vi "rotina de aquisição dos dados de caracterização.vi"() -> ()   [LabVIEW 2011]
uses:
  <vilib>/express/express analysis/Spectral/XNode/ExpressSpectralMeasurementsBlockNode.xnode
  <vilib>/express/express analysis/Spectral/Block/exnSpectralBlock spectral measurements power poly.vi
  <vilib>/express/express analysis/Spectral/Block/exnSpectralBlock spectral measurements power DDT.vi
  <vilib>/express/express analysis/Spectral/Block/exnSpectralBlock spectral measurements power WFM.vi
panel:
  out "Power Spectrum":cluster{"f0":dbl, "df":dbl, "magnitude":dbl[]}(graph)
  in  "Upper Cut-Off":dbl=65.0
  out "Waveform Graph":dynamicdata(graph)
  in  "Frequência de Corte (Hz)":dbl=60.0 caption="Lower Cut-Off"
  out "Gráfico - tempo real/sinal bruto":dbl[](graph) caption="Gráfico - tempo real/bruto"
  in  "stop":bool
  out "Gráfico - tempo real/sinal filtrado":dbl[](graph) caption="Gráfico - tempo real/filtrado"
  out "Gráfico 2":waveform(dbl)(graph)
  in  "Parar programa":bool
  in  "OK Button":bool
  out "direito":dbl
  out "esquerdo":dbl
  # "PROGRAMA DE AQUISIÇÃO DE SINAL PARA CARACTERIZAÇÃO"
  # "SINAL AQUISITADO EM TEMPO REAL"
  # "SINAL A SER GRAVADO PARA PROCESSAMENTO"
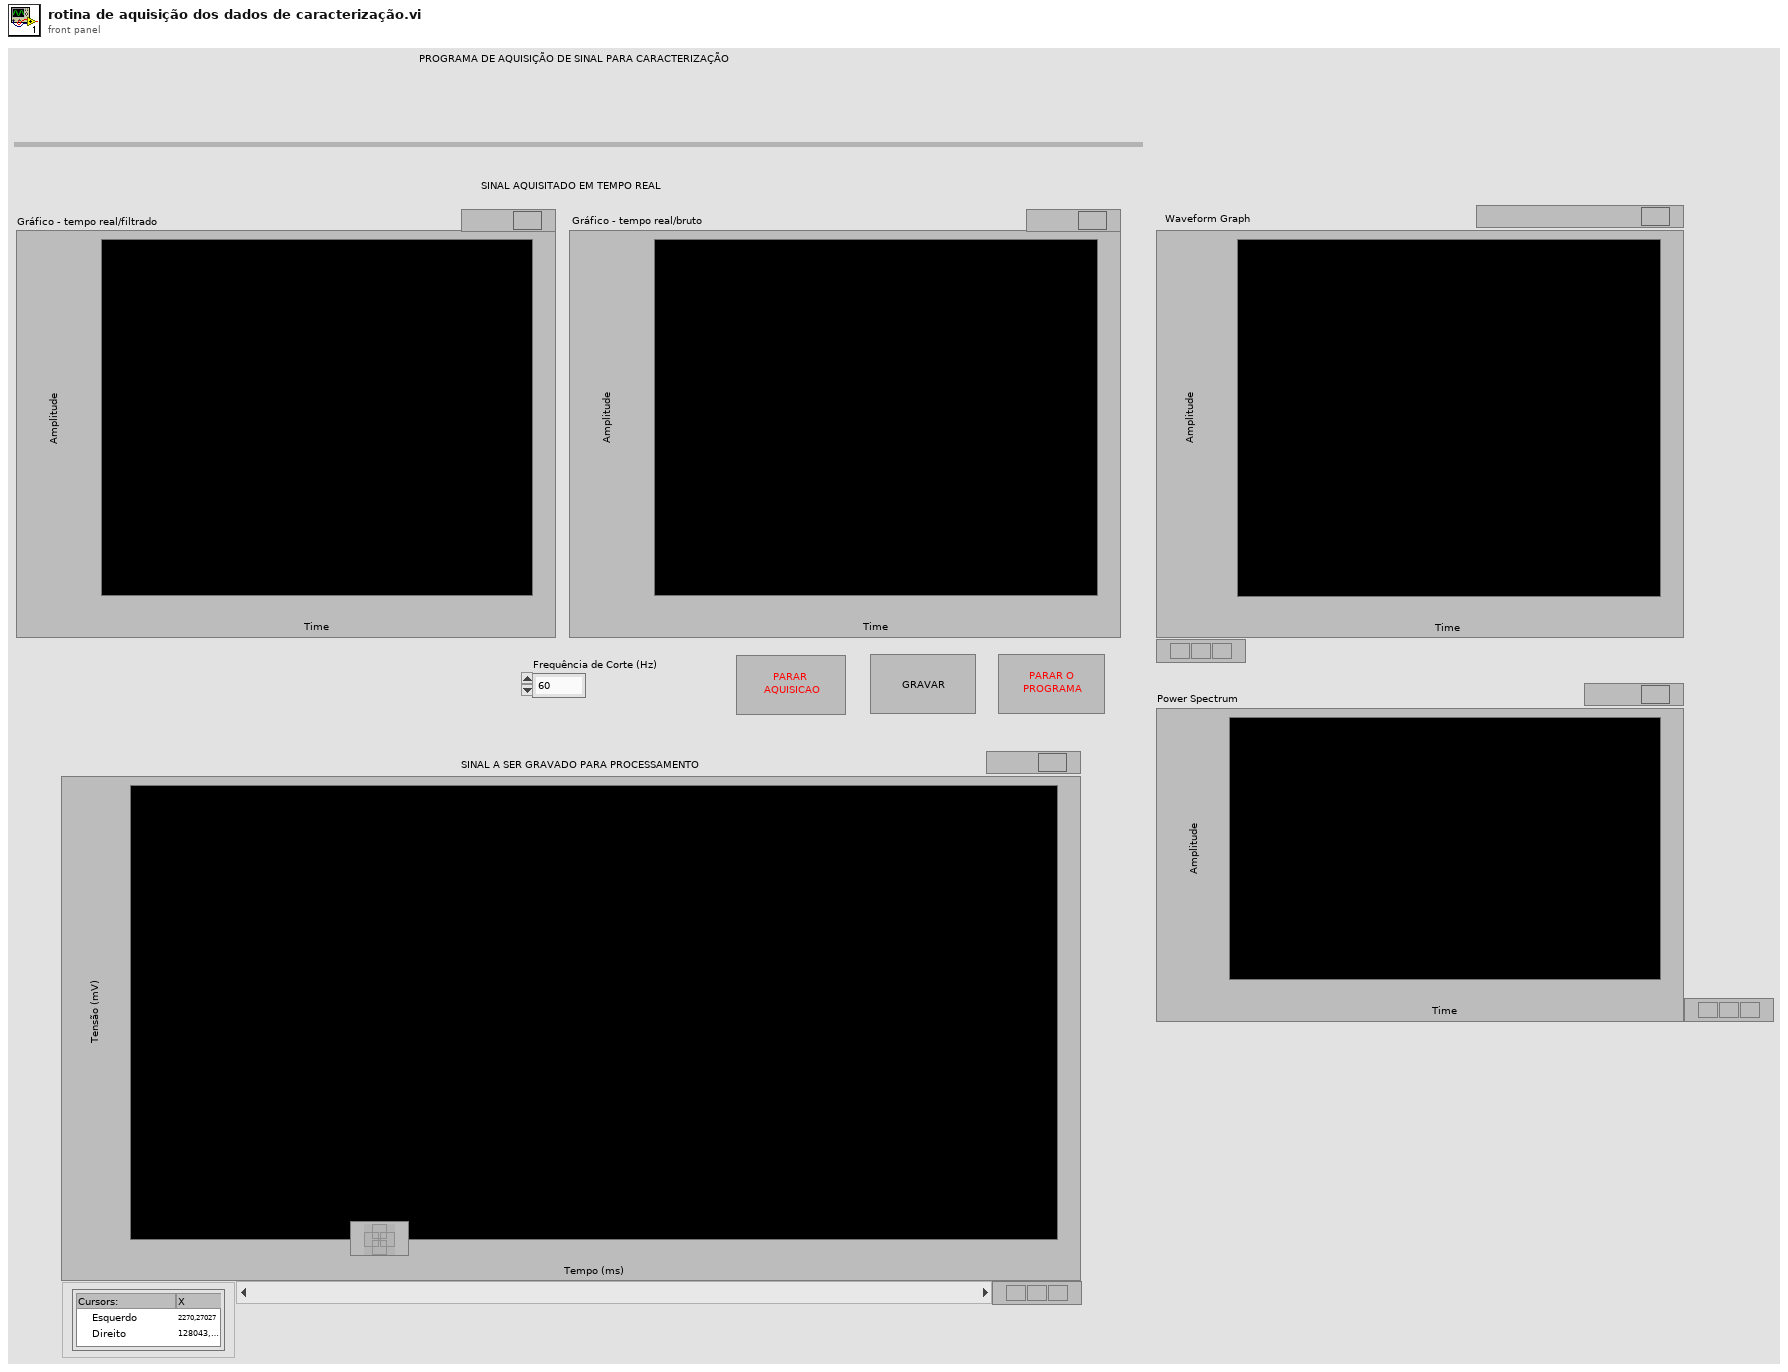
[diagram p1: front panel]
types:
  T1 = cluster{"averaging mode":u16, "weighting mode":u16, "number of averages":u32}
  T2 = cluster{"dB On (F)":bool, "unwrap phase (F)":bool, "convert to degree (F)":bool}
  T3 = typedef "NI_Matrix.lvlib/RealMatrix.ctl" = dbl[][]
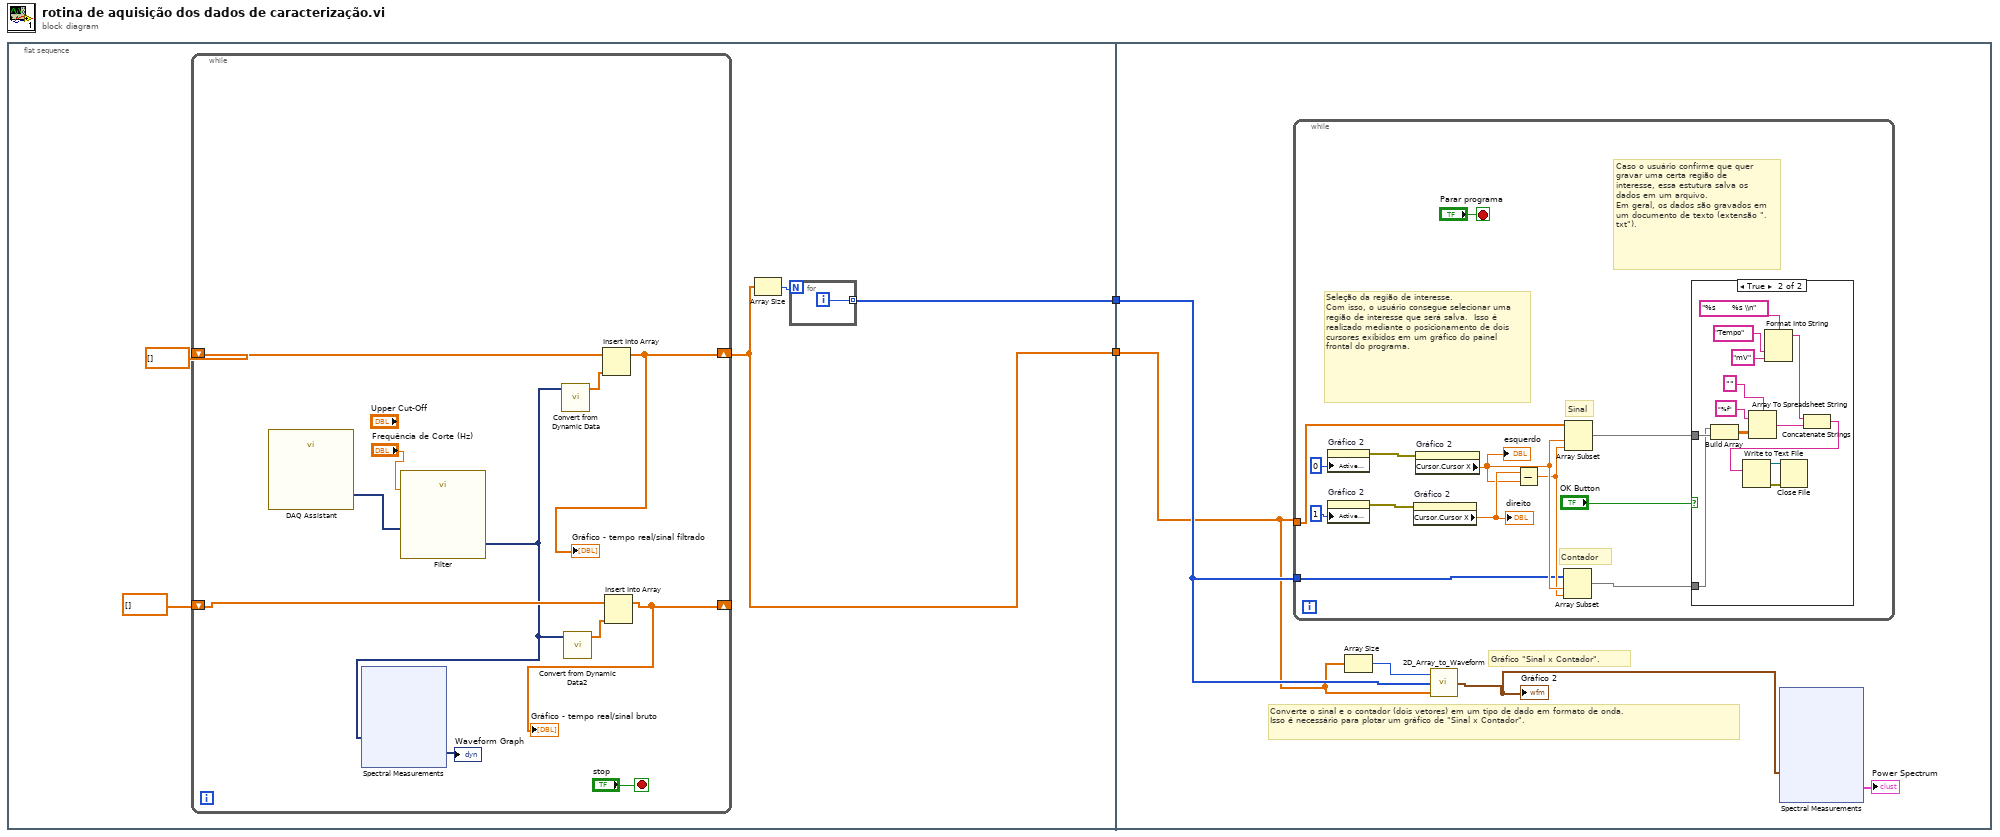
[diagram p0: block diagram]
diagram:
  n1 = flat-sequence {
    tunnel: [w5] -> w2
    tunnel: [w3] -> w1
    tunnel: w2 -> [w32]
    tunnel: w1 -> [w31]
    frame #0 {
      n2 = while {
        shift-right: [w16] -> w3
        shift-left: dbl[] [] ("Array") -> [w18]
        shift-right: [w13] -> _
        shift-left: dbl[] [] ("Array") -> [w14]
        stop <- "stop" stop-if-true
        n3 = call "DAQ Assistant"() -> ("data"=w11:dynamicdata)  [unwired: 16 in, 3 out]
        n4 = call "Filter"("Lower Cut-Off"="Frequência de Corte (Hz)", "Signal"=w11) -> ("Filtered Signal"=w10:dynamicdata)  [unwired: 8 in, 1 out]
        n5 = xnode "Spectral Measurements"("Signals"=w10) -> ("Power Spectrum"=→"Waveform Graph":dynamicdata)  [unwired: 1 in, 1 out]
        n6 = call "Convert from Dynamic Data"("Dynamic Data Type"=w10) -> ("Array"=w19:dbl[])  [unwired: 3 in]
        n7 = call "Convert from Dynamic Data2"("Dynamic Data Type"=w10) -> ("Array"=w15:dbl[])  [unwired: 3 in]
        n8 = Insert Into Array(array=w18, new element=w19) -> (w16:dbl[])  [unwired: 1 in]
        "Gráfico - tempo real/sinal filtrado" <- w16
        n9 = Insert Into Array(array=w14, new element=w15) -> (w13:dbl[])  [unwired: 1 in]
        "Gráfico - tempo real/sinal bruto" <- w13
      }
      n10 = Array Size(array=w3) -> (size(s)=w6:i32)
      n11 = for {
        N: w6 -> [_]
        tunnel: [w8] -> w5 mode=indexing
        i -> [w8]
      }
    }
    frame #1 {
      # "Gráfico \"Sinal x Contador\"."
      # "Converte o sinal e o contador (dois vetores) em um tipo de dado em formato de onda. \nIsso é necessário para plotar um gráfico de \"Sinal x Contador\"."
      n12 = while {
        tunnel: w32 -> [w45]
        tunnel: w31 -> [w43]
        stop <- "Parar programa" stop-if-true
        # "Caso o usuário confirme que quer gravar uma certa região de interesse, essa estutura salva os dados em um arquivo.\nEm geral, os dados são gravados em um documento de texto (extensão \".txt\")."
        # "Seleção da região de interesse. \nCom isso, o usuário consegue selecionar uma região de interesse que será salva.  Isso é realizado mediante o posicionamento de dois cursores exibidos em um gráfico do painel frontal do programa."
        # "Contador"
        # "Sinal"
        n13 = property on="Gráfico 2" class="WFGraph (strict)"("Active Cursor"=u32 0) -> (error out=w55:errorcluster)  [unwired: 2 in, 1 out]
        n14 = property on="Gráfico 2" class="WFGraph (strict)"("Active Cursor"=u32 1) -> (error out=w53:errorcluster)  [unwired: 2 in, 1 out]
        n15 = property on="Gráfico 2" class="WFGraph (strict)"(error in=w53) -> ("Cursor.Cursor X"=w51:dbl)  [unwired: 1 in, 2 out]
        "direito" <- w51
        n16 = property on="Gráfico 2" class="WFGraph (strict)"(error in=w55) -> ("Cursor.Cursor X"=w47:dbl)  [unwired: 1 in, 2 out]
        "esquerdo" <- w47
        n17 = Subtract(x=w51, y=w47) -> (x-y=w46:dbl)
        n18 = Array Subset(array=w45, index=w47, length=w46) -> (w44:i32[])
        n19 = Array Subset(array=w43, index=w47, length=w46) -> (w49:dbl[])
        n20 = case shown="True" "OK Button" {
          tunnel: w49 -> [_ w57]
          tunnel: w44 -> [_ w56]
          frame False {
          }
          frame True {
            n21 = Build Array(w56, w57) -> (w61:T3)
            n22 = Array To Spreadsheet String(delimiter (Tab)="", array=w61, 3:"%f" ("format string")) -> (spreadsheet string=w63:string)
            n23 = Format Into String(format string="%s        %s \\n", "Tempo" ("input 1"), "mV" ("input 2")) -> (resulting string=w62:string)  [unwired: 2 in, 1 out]
            n24 = Concatenate Strings(w62, w63) -> (w58:string)
            n25 = Write to Text File(text=w58) -> (refnum out=w60:refnum<file>, error out=w59:errorcluster)  [unwired: 3 in, 1 out]
            n26 = Close File(refnum=w60, error in=w59) -> ()  [unwired: 2 out]
          }
        }
      }
      n27 = Array Size(array=w31) -> (size(s)=w33:i32)
      n28 = call "2D_Array_to_Waveform.vi"("Y"=w31, "X"=w32, "Nº de amostras"=w33) -> ("output waveform"=w30:waveform(dbl))
      "Gráfico 2" <- w30
      n29 = xnode "Spectral Measurements"("Signals"=w30) -> ("Power Spectrum"=→"Power Spectrum":cluster{"f0":dbl, "df":dbl, "magnitude":dbl[]})  [unwired: 1 in, 1 out]
    }
  }
